vi "Get Relay Info.vi"(8 "error in (no error)":errorcluster, 10 "relay string":string, 11 "Route Manager in":refnum<class "Route Manager.lvclass">) -> (0 "error out":errorcluster, 2 "relay info":T1)   [LabVIEW 2015, in "Route Manager.lvclass"]
uses:
  Route Manager.lvclass
  Relay Info.ctl
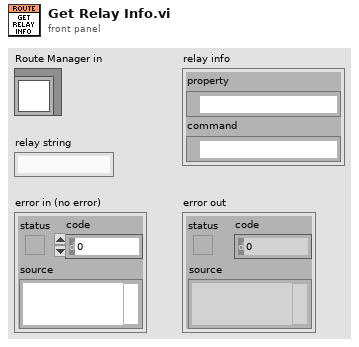
[diagram p1: front panel]
types:
  T1 = typedef "Route Manager.lvclass/Relay Info.ctl" = cluster{"property":refnum<k21>, "command":refnum<k21>}
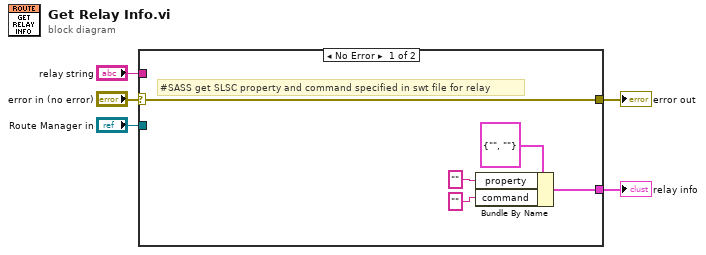
[diagram p0: block diagram]
diagram:
  n1 = case shown="No Error" "error in (no error)" {
    selector: "error in (no error)" -> [w10 w11]
    tunnel: [w10 w11] -> w4
    tunnel: "Route Manager in" -> [_ _]
    tunnel: [w9 _] -> w2
    tunnel: "relay string" -> [_ _]
    frame No Error {
      # "#SASS get SLSC property and command specified in swt file for relay"
      n2 = Bundle By Name(cluster=T1 {"property"="", "command"=""} ("relay info"), "property"="", "command"="") -> (w9:T1)
    }
    frame Error {
    }
  }
  "error out" <- w4
  "relay info" <- w2
